vi "Module Template SM.vi"(8 "error in (no error)":errorcluster, 11 "Module_Refs":T1={"ModuleName"=enum."Controller", "Queue"=refnum, "user event"=refnum, "VI Refnum"=refnum, "ShowFP"=FALSE, "StatesTracking Enabled"=FALSE}) -> (0 "error out":errorcluster)   [LabVIEW 2021, in "Architecture.lvlib"]
doc: "Main Module Template of the architecture. Use this as a template to integrate new independent processes into your application."
uses:
  Architecture.lvlib
  Typedefs/Enum_Module_Name.ctl
  Typedefs/Message.ctl
  Typedefs/Module References.ctl
  Typedefs/State Machine Data.ctl
  Typedefs/Application Configuration.ctl
  Modules/Module Template/SubVIs/Module Template Configuraton Extractor API.vi
panel:
  in  "Stop App":bool
  out "Message":string
  in  "Stop Module":bool
  # "#Architecture\n\nPlace inside this box all visible data."
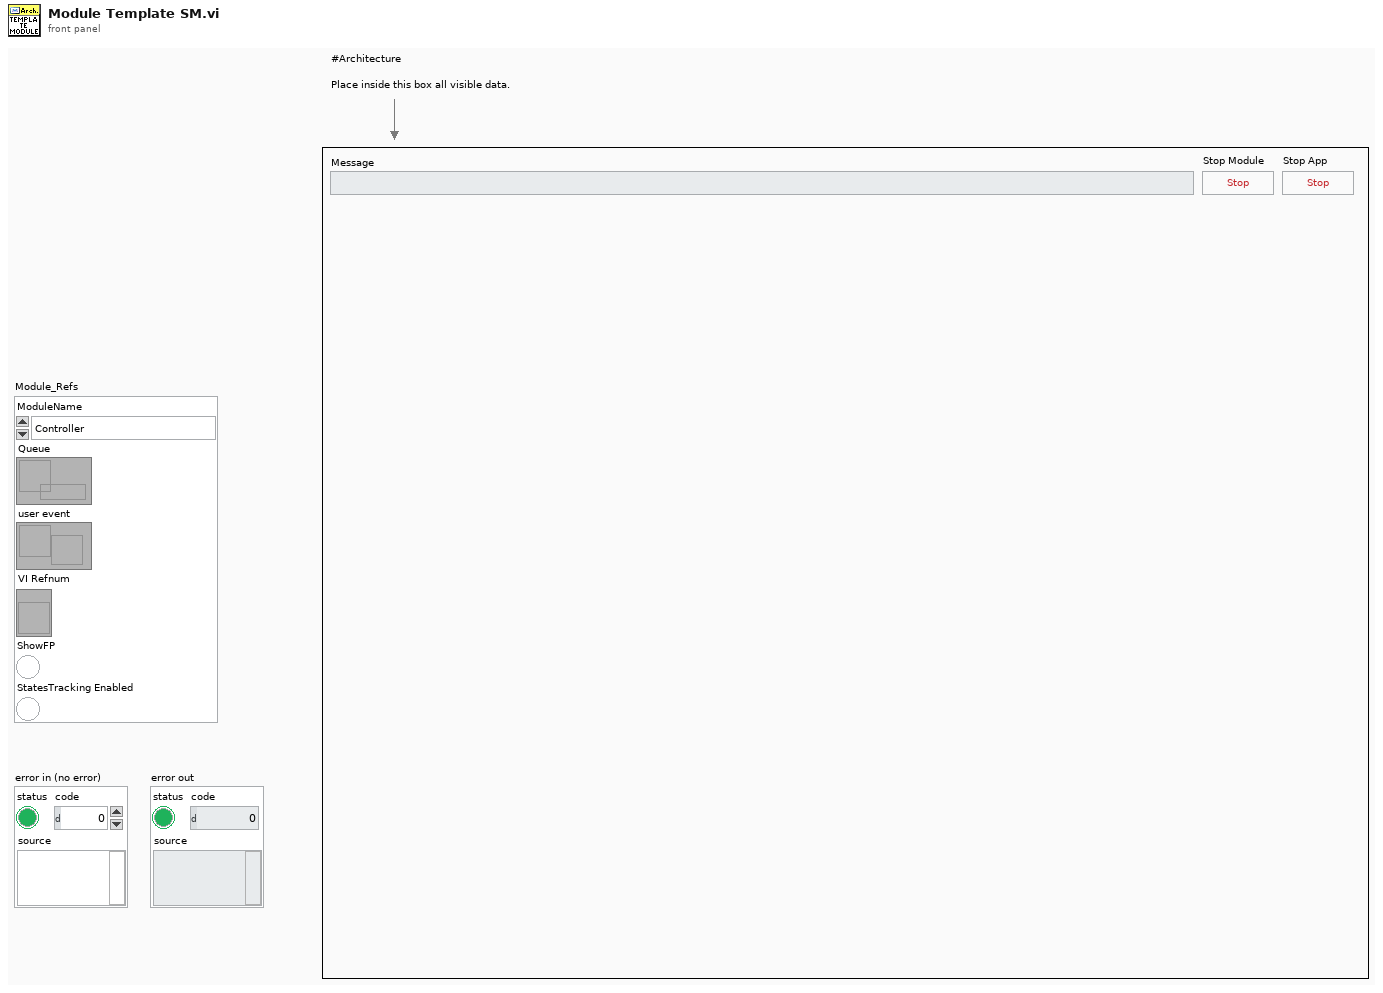
[diagram p1: front panel]
types:
  T1 = typedef "Architecture.lvlib/Module References.ctl" = cluster{"ModuleName":T2, "Queue":refnum<queue>, "user event":refnum<user-event>, "VI Refnum":refnum<vi>, "ShowFP":bool, "StatesTracking Enabled":bool}
  T2 = typedef "Architecture.lvlib/Enum_Module_Name.ctl" = enum16{"Configuration", "Error_Handler", "Log", "Database", "Controller"}
  T3 = typedef "Architecture.lvlib/State Machine Data.ctl" = cluster{"Module_Refs":T1, "Response Data":variant, "Module Template Config":T4}
  T4 = typedef "Architecture.lvlib/Config.ctl" = cluster{"Module Enabled":bool}
  T5 = enum32{"Invalid", "Standard", "Closed", "Hidden", "Minimized", "Maximized"}
  T6 = typedef "Error_Manager.lvlib/LogRotate.lvclass/LogData.ctl" = cluster{"error in":errorcluster, "replacements":string[], "Time Stamp":timestamp}
  T7 = typedef "Architecture.lvlib/Module Template.lvlib/Config.ctl" = cluster{"Module Enabled":bool}
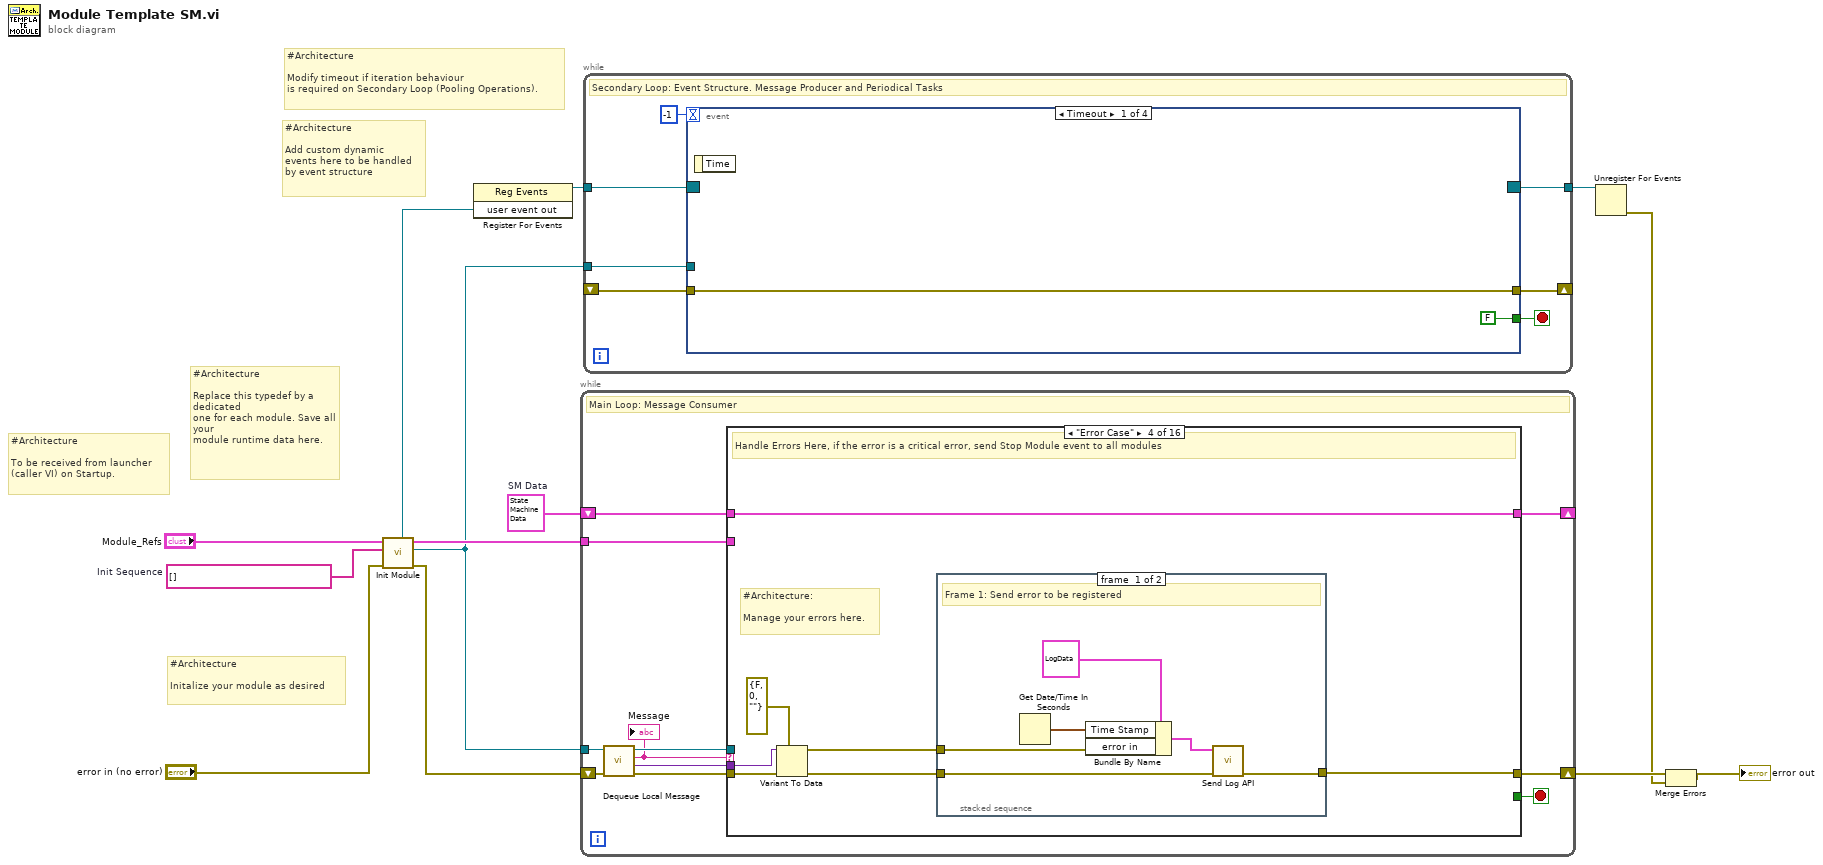
[diagram p0: block diagram]
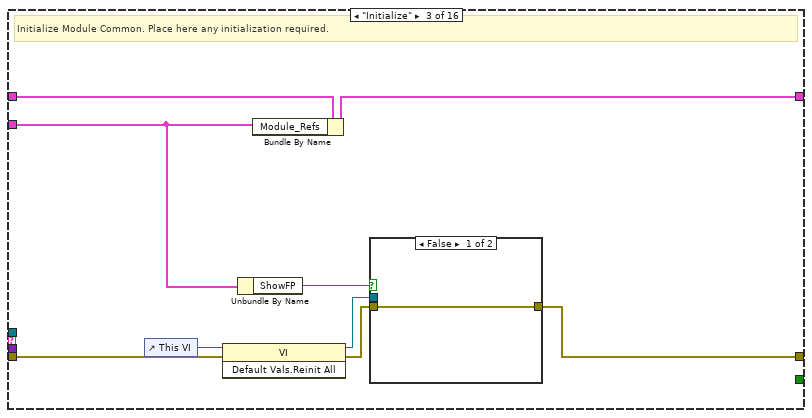
[diagram p4: hidden frame]
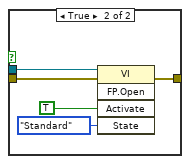
[diagram p5: hidden frame]
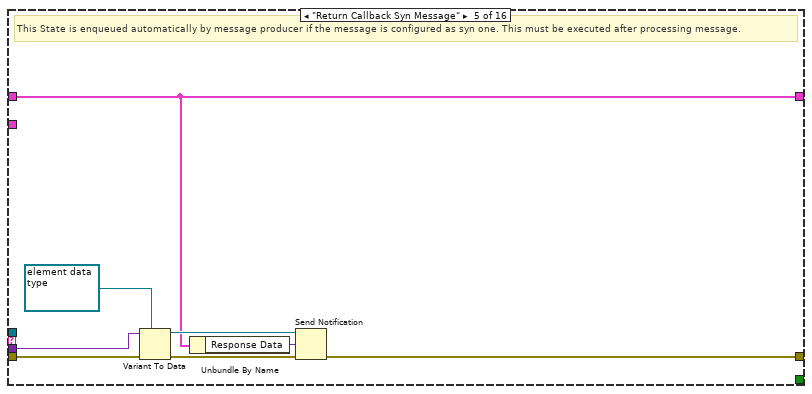
[diagram p8: hidden frame]
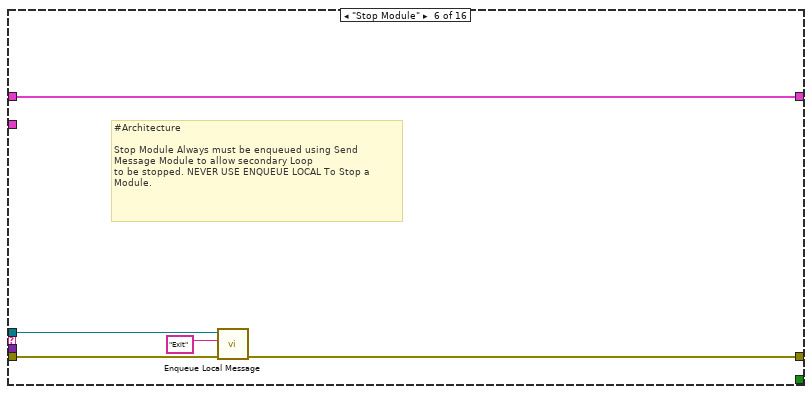
[diagram p9: hidden frame]
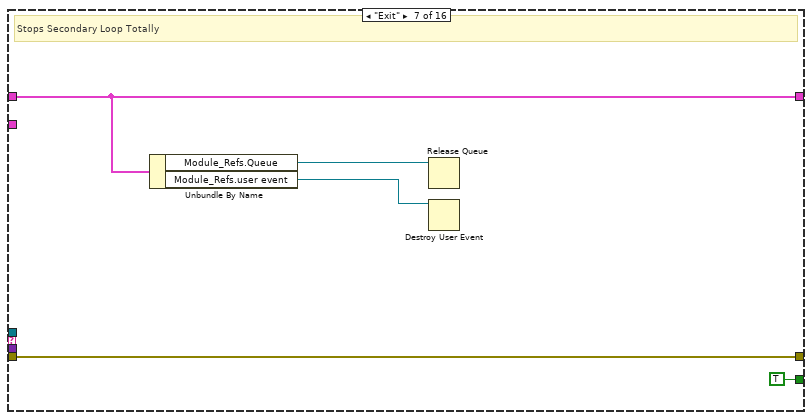
[diagram p10: hidden frame]
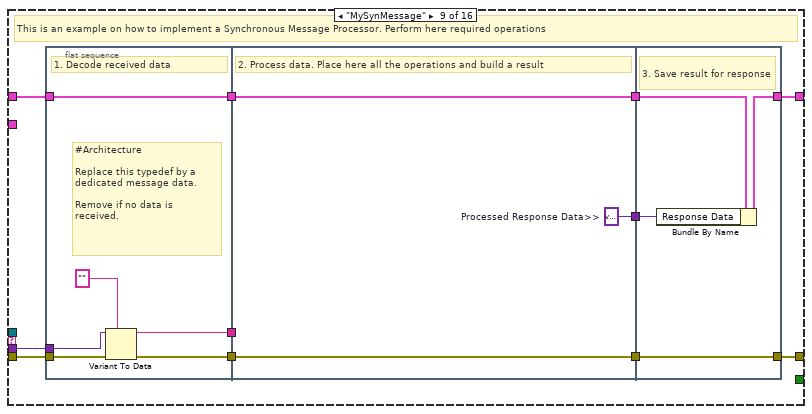
[diagram p12: hidden frame]
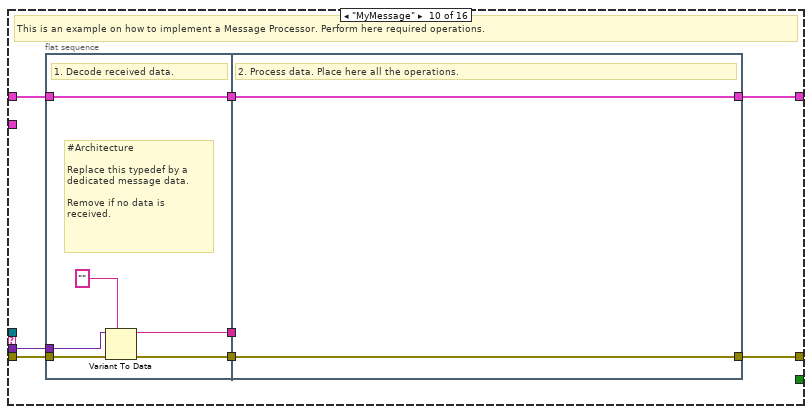
[diagram p13: hidden frame]
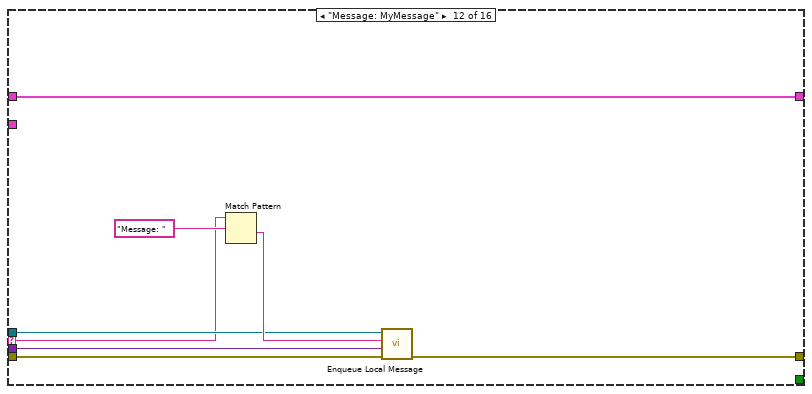
[diagram p15: hidden frame]
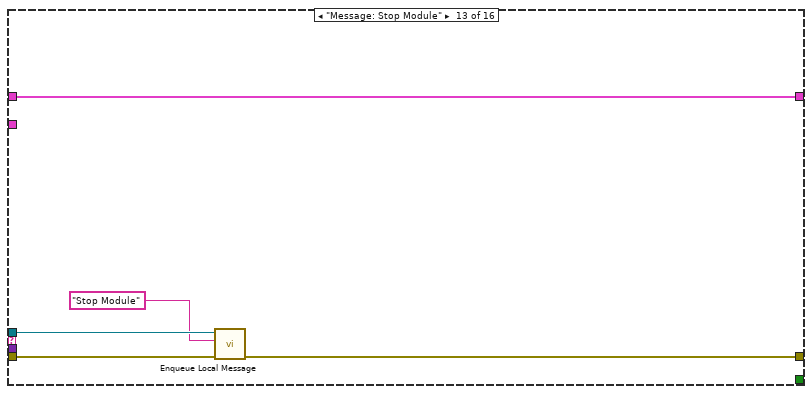
[diagram p16: hidden frame]
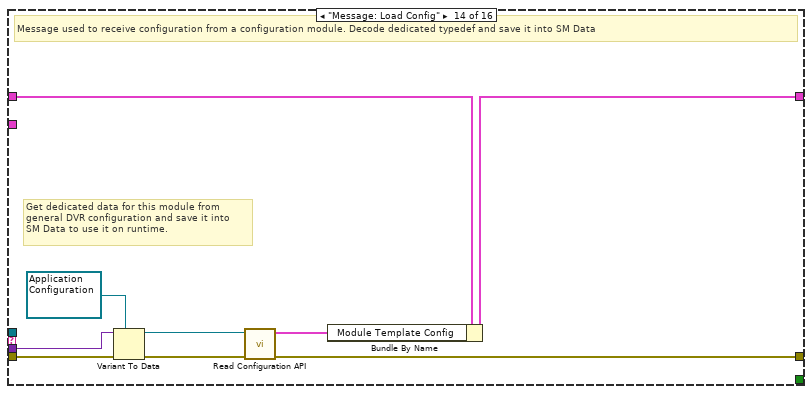
[diagram p17: hidden frame]
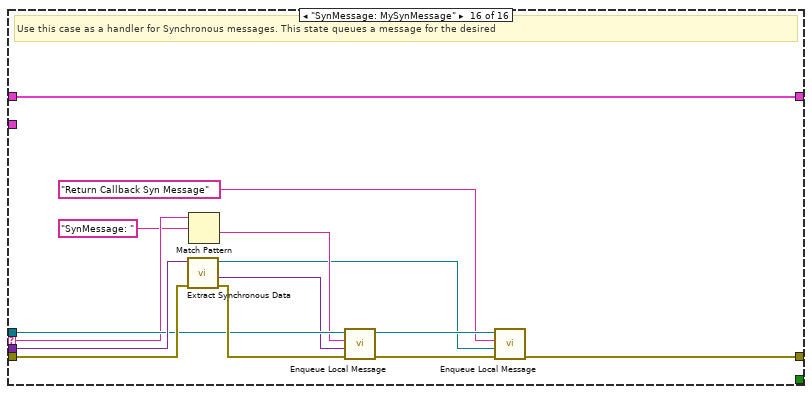
[diagram p19: hidden frame]
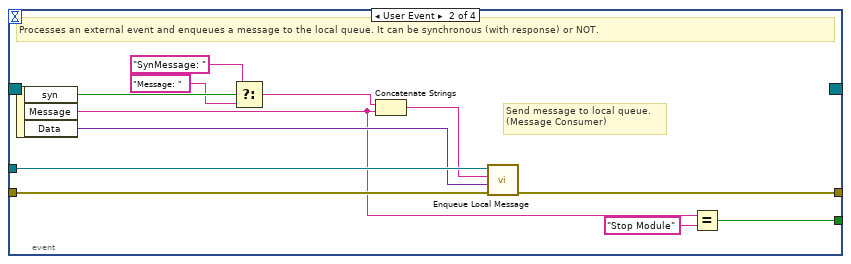
[diagram p20: hidden frame]
diagram:
  w10 = string[] []  # Init Sequence
  w13 = T3 {"Module_Refs"={"ModuleName"=enum."Controller", "Queue"=refnum, "user event"=refnum, "VI Refnum"=refnum, "ShowFP"=FALSE, "StatesTracking Enabled"=FALSE}, "Response Data"=variant, "Module Template Config"={"Module Enabled"=FALSE}}  # SM Data
  # "#Architecture\n\nModify timeout if iteration behaviour \nis required on Secondary Loop (Pooling Operations)."
  # "#Architecture\n\nAdd custom dynamic \nevents here to be handled \nby event structure"
  # "#Architecture\n\nInitalize your module as desired"
  # "#Architecture\n\nTo be received from launcher \n(caller VI) on Startup."
  # "#Architecture\n\nReplace this typedef by a dedicated \none for each module. Save all your \nmodule runtime data here."
  n1 = call "Init Module.vi"("error in (no error)"="error in (no error)", "Init Sequence"=w10, "Module Refs"="Module_Refs") -> ("error out"=w12:errorcluster, "queue out"=w1:refnum<queue>, "Module Refs Out"=w3:T1, "user event out"=w2:refnum<user-event>)  [unwired: 5 in]
  n2 = register-events(w2) -> (reference out=w9:refnum<event-registration>)  [unwired: 2 in, 1 out]
  n3 = while {
    shift-right: [w23] -> _
    shift-left: w13 -> [w24]
    shift-right: [w22] -> w7
    shift-left: w12 -> [w20]
    tunnel: w1 -> [w21]
    tunnel: w3 -> [w14]
    stop <- w15 stop-if-true
    # "Main Loop: Message Consumer"
    n4 = call "Dequeue Local Message.vi"("error in"=w20, "Msg queue in"=w21) -> ("error out"=w19:errorcluster, "Data"=w16:variant, "Message"=w17:string, "queue out"=w18:refnum<queue>)  [unwired: 6 in]
    "Message" <- w17
    n5 = case shown="\"Error Case\"" w17 {
      selector: w17 -> [_ _ _ _ _ _ _ _ _ _ _ w123 _ _ _ w155]
      tunnel: w24 -> [w26 w28 w37 w50 w62 w73 w76 w80 w91 w112 w122 w130 w135 w144 w146 w160]
      tunnel: [w26 w28 w35 w50 w62 w73 w76 w80 w90 w105 w122 w130 w135 w137 w146 w160] -> w23
      tunnel: w19 -> [w25 w27 w36 w49 w68 w72 w78 w79 w84 w108 w121 w127 w134 w143 w145 w159]
      tunnel: [w25 w27 w31 w45 w67 w71 w78 w79 w89 w111 w121 w124 w133 w138 w145 w149] -> w22
      tunnel: w18 -> [_ _ _ _ _ w70 _ _ _ _ _ w125 w132 _ _ w156]
      tunnel: w16 -> [_ _ _ w48 w65 _ _ _ w83 w107 _ w126 _ w142 _ w157]
      tunnel: [_ _ _ _ _ _ TRUE _ _ _ _ _ _ _ _ _] -> w15
      tunnel: w14 -> [_ _ w34 _ _ _ _ _ _ _ _ _ _ _ _ _]
      frame "--------State Machine Arquitechture Operations--------" {
      }
      frame "Idle", Default {
        # "Use this state to make iterations if required."
      }
      frame "Initialize" {
        # "Initialize Module Common. Place here any initialization required."
        n6 = control-ref of="This VI"() -> (w29:refnum<vi>)
        n7 = invoke class="VI" method="Default Vals.Reinit All"(reference=w29, error in=w36) -> (reference out=w32:refnum<vi>, error out=w33:errorcluster)  [unwired: 1 in, 1 out]
        n8 = Unbundle By Name(w34) -> ("ShowFP"=w30:bool)
        n9 = Bundle By Name(cluster=w37, "Module_Refs"=w34) -> (w35:T3)
        n10 = case shown="False" w30 {
          tunnel: w33 -> [w38 w43]
          tunnel: [w38 w42] -> w31
          tunnel: w32 -> [_ w41]
          frame False {
          }
          frame True {
            n11 = invoke class="VI" method="FP.Open"(reference=w41, error in=w43, "Activate"=TRUE ("Activate?"), "State"=T5."Standard") -> (error out=w42:errorcluster)  [unwired: 1 in, 4 out]
          }
        }
      }
      frame "Error Case" {
        # "#Architecture: \n\nManage your errors here."
        # "Handle Errors Here, if the error is a critical error, send Stop Module event to all modules"
        n12 = Variant To Data(error in=w49, type=errorcluster {"status"=FALSE, "code"=0, "source"=""} ("error constant"), Variant=w48) -> (data=w44:errorcluster, error out=w46:errorcluster)
        n13 = stacked-sequence {
          tunnel: w46 -> [w56 w58]
          tunnel: [w55 _] -> w45
          tunnel: w44 -> [w53 w57]
          frame #0 {
            # "Frame 1: Send error to be registered"
            n14 = Get Date/Time In Seconds() -> (seconds since 1Jan1904=w52:timestamp)
            n15 = Bundle By Name(cluster=T6 {"error in"={"status"=FALSE, "code"=0, "source"=""}, "replacements"=[], "Time Stamp"=timestamp(0 s since 1904-01-01)} ("Data"), "Time Stamp"=w52, "error in"=w53) -> (w51:T6)
            n16 = call "Send Log API.vi"("error in (no error)"=w56, "Data"=w51) -> ("error out"=w55:errorcluster)  [unwired: 9 in]
          }
          frame #1 {
            # "Frame 2: Manage your errors here"
            n17 = case shown="No Error" w57 {
              tunnel: [w59 w60] -> _
              tunnel: w58 -> [w59 w60]
              frame No Error {
              }
              frame Error {
                # "#Architecture \n\nPlace here critical errors to be managed \nin the desired way."
              }
            }
          }
        }
      }
      frame "Return Callback Syn Message" {
        # "This State is enqueued automatically by message producer if the message is configured as syn one. This must be executed after processing message."
        n18 = Variant To Data(error in=w68, type=refnum<notifier> refnum ("notifier out"), Variant=w65) -> (data=w63:refnum<notifier>, error out=w66:errorcluster)
        n19 = Unbundle By Name(w62) -> ("Response Data"=w61:variant)
        n20 = Send Notification(notification=w61, notifier=w63, error in (no error)=w66) -> (error out=w67:errorcluster)  [unwired: 1 out]
      }
      frame "Stop Module" {
        # "#Architecture\n\nStop Module Always must be enqueued using Send Message Module to allow secondary Loop\nto be stopped. NEVER USE ENQUEUE LOCAL To Stop a Module."
        n21 = call "Enqueue Local Message.vi"("error in"=w72, "Message"="Exit", "Msg queue in"=w70) -> ("error out"=w71:errorcluster)  [unwired: 7 in, 1 out]
      }
      frame "Exit" {
        # "Stops Secondary Loop Totally"
        n22 = Unbundle By Name(w76) -> ("Module_Refs.Queue"=w75:refnum<queue>, "Module_Refs.user event"=w74:refnum<user-event>)
        n23 = Release Queue(queue=w75) -> ()  [unwired: 2 in, 3 out]
        n24 = Destroy User Event(user event=w74) -> ()  [unwired: 1 in, 1 out]
      }
      frame "--------------State Machine Custom States-------------" {
      }
      frame "MySynMessage" {
        # "This is an example on how to implement a Synchronous Message Processor. Perform here required operations"
        n25 = flat-sequence {
          tunnel: w84 -> [w95]
          tunnel: w91 -> [w97]
          tunnel: [w97] -> w88
          tunnel: [w93] -> w87
          tunnel: w83 -> [w94]
          tunnel: [w92] -> w82
          tunnel: w88 -> [w100]
          tunnel: w87 -> [w99]
          tunnel: [w100] -> w86
          tunnel: [w99] -> w85
          tunnel: w82 -> [_]
          tunnel: [w98] -> w81
          tunnel: [w103] -> w89
          tunnel: [w102] -> w90
          tunnel: w86 -> [w104]
          tunnel: w85 -> [w103]
          tunnel: w81 -> [w101]
          frame #0 {
            # "#Architecture\n\nReplace this typedef by a dedicated message data.\n\nRemove if no data is received."
            # "1. Decode received data"
            n26 = Variant To Data(error in=w95, type="", Variant=w94) -> (data=w92:string, error out=w93:errorcluster)
          }
          frame #1 {
            w98 = variant  # Processed Response Data>>
            # "2. Process data. Place here all the operations and build a result"
          }
          frame #2 {
            # "3. Save result for response"
            n27 = Bundle By Name(cluster=w104, "Response Data"=w101) -> (w102:T3)
          }
        }
      }
      frame "MyMessage" {
        # "This is an example on how to implement a Message Processor. Perform here required operations."
        n28 = flat-sequence {
          tunnel: w108 -> [w116]
          tunnel: w112 -> [w118]
          tunnel: [w118] -> w110
          tunnel: [w114] -> w109
          tunnel: w107 -> [w115]
          tunnel: [w113] -> w106
          tunnel: w110 -> [w119]
          tunnel: w109 -> [w120]
          tunnel: w106 -> [_]
          tunnel: [w120] -> w111
          tunnel: [w119] -> w105
          frame #0 {
            # "#Architecture\n\nReplace this typedef by a dedicated message data.\n\nRemove if no data is received."
            # "1. Decode received data."
            n29 = Variant To Data(error in=w116, type="", Variant=w115) -> (data=w113:string, error out=w114:errorcluster)
          }
          frame #1 {
            # "2. Process data. Place here all the operations."
          }
        }
      }
      frame "--------------Dynamic Events Messages----------------" {
      }
      frame "Message: MyMessage" {
        n30 = Match Pattern(string=w123, regular expression="Message: ") -> (after substring=w128:string)  [unwired: 1 in, 3 out]
        n31 = call "Enqueue Local Message.vi"("error in"=w127, "Data"=w126, "Message"=w128, "Msg queue in"=w125) -> ("error out"=w124:errorcluster)  [unwired: 6 in, 1 out]
      }
      frame "Message: Stop Module" {
        n32 = call "Enqueue Local Message.vi"("error in"=w134, "Message"="Stop Module", "Msg queue in"=w132) -> ("error out"=w133:errorcluster)  [unwired: 7 in, 1 out]
      }
      frame "Message: Load Config" {
        # "Get dedicated data for this module from \ngeneral DVR configuration and save it into \nSM Data to use it on runtime."
        # "Message used to receive configuration from a configuration module. Decode dedicated typedef and save it into SM Data"
        n33 = Variant To Data(error in=w143, type=refnum<data-value> refnum ("data value reference"), Variant=w142) -> (data=w140:refnum<data-value>, error out=w139:errorcluster)
        n34 = call-poly "Read Configuration API.vi"("error constant"=w139, "General Config DVR In"=w140) -> ("error out"=w138:errorcluster, "Module Template Config"=w136:T7)  [unwired: 8 in]
        n35 = Bundle By Name(cluster=w144, "Module Template Config"=w136) -> (w137:T3)
      }
      frame "------------Synchronous Event Messages--------------" {
      }
      frame "SynMessage: MySynMessage" {
        # "Use this case as a handler for Synchronous messages. This state queues a message for the desired"
        n36 = call "Extract Synchronous Data.vi"("error in 2"=w159, "Variant"=w157) -> ("error in"=w158:errorcluster, "Data Out"=w152:variant, "notifier out"=w147:refnum<notifier>)  [unwired: 7 in]
        n37 = Match Pattern(string=w155, regular expression="SynMessage: ") -> (after substring=w153:string)  [unwired: 1 in, 3 out]
        n38 = call "Enqueue Local Message.vi"("error in"=w158, "Data"=w152, "Message"=w153, "Msg queue in"=w156) -> ("error out"=w151:errorcluster, "queue out"=w150:refnum<queue>)  [unwired: 6 in]
        n39 = call "Enqueue Local Message.vi"("error in"=w151, "Data"=w147, "Message"="Return Callback Syn Message", "Msg queue in"=w150) -> ("error out"=w149:errorcluster)  [unwired: 6 in, 1 out]
      }
    }
  }
  n40 = while {
    tunnel: w9 -> [w167]
    tunnel: w1 -> [w164]
    tunnel: [w163] -> w8
    shift-right: [w161] -> _
    shift-left: _ -> [w162]
    stop <- w165 stop-if-true
    # "Secondary Loop: Event Structure. Message Producer and Periodical Tasks"
    n41 = event shown="[0] Timeout" {
      selector: w167 -> [_ _ _ _]
      dyn-events: [_ _ _ _] -> w163
      timeout: -1 -> [_ _ _ _]
      tunnel: [FALSE w176 TRUE _] -> w165
      tunnel: w164 -> [_ w181 w183 _]
      tunnel: w162 -> [w168 w180 w186 w188]
      tunnel: [w168 w179 w184 w187] -> w161
      event Timeout {
        n42 = event-data() -> ()  [unwired: 1 in, 1 out]
      }
      event User Event {
        # "Send message to local queue. \n(Message Consumer)"
        # "Processes an external event and enqueues a message to the local queue. It can be synchronous (with response) or NOT."
        n43 = event-data() -> ("syn"=w173:bool, "Message"=w175:string, "Data"=w178:variant)  [unwired: 1 in]
        n44 = Select(t="SynMessage: " ("string"), s=w173, f="Message: " ("string")) -> (s? t:f=w170:string)
        n45 = Concatenate Strings(w170, w175) -> (w177:string)
        n46 = call "Enqueue Local Message.vi"("error in"=w180, "Data"=w178, "Message"=w177, "Msg queue in"=w181) -> ("error out"=w179:errorcluster)  [unwired: 6 in, 1 out]
        n47 = Equal?(x=w175, y="Stop Module") -> (x = y?=w176:bool)
      }
      event "Stop Module": Value Change {
        n48 = event-data() -> ()  [unwired: 1 in, 1 out]
        n49 = call "Enqueue Local Message.vi"("error in"=w186, "Message"="Stop Module", "Msg queue in"=w183) -> ("error out"=w184:errorcluster)  [unwired: 7 in, 1 out]
      }
      event "Stop App": Value Change {
        w190 = TRUE  # All Modules
        # "Send Stop To All Modules"
        n50 = event-data() -> ()  [unwired: 1 in, 1 out]
        n51 = call "Send Message Modules.vi"("All Modules"=w190, "Error In"=w188, "Message"="Stop Module") -> ("error in (no error)"=w187:errorcluster)  [unwired: 8 in]
      }
    }
  }
  n52 = Unregister For Events(event registration refnum=w8) -> (error out=w6:errorcluster)  [unwired: 1 in]
  n53 = Merge Errors(w7, w6) -> (→"error out":errorcluster)
